vi "Unit Test.vi"() -> ()   [LabVIEW 2018]
uses:
  Force Test Stand.lvclass
  Force Test Stand.lvclass/Force Test Stand.ctl
panel:
  out "error out":errorcluster
  in  "error in (no error)":errorcluster
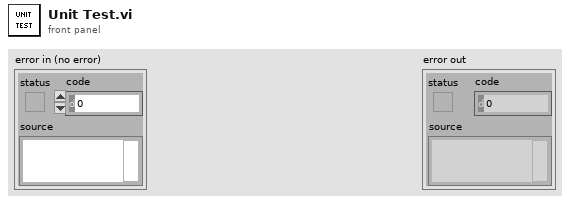
[diagram p1: front panel]
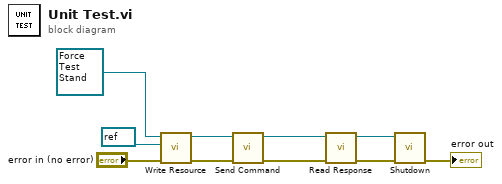
[diagram p0: block diagram]
diagram:
  n1 = call "Write Resource.vi"("error in (no error)"="error in (no error)", "Resource"=refnum<visa-resource-name> refnum, "Force Test Stand in"=refnum<class "Force Test Stand.lvclass"> refnum) -> ("error out"=w1:errorcluster, "Force Test Stand out"=w2:refnum<class "Force Test Stand.lvclass">)  [unwired: 7 in]
  n2 = call-dynamic "Send Command.vi"("error in (no error)"=w1, "Force Test Stand in"=w2) -> ("error out"=w5:errorcluster, "Force Test Stand out"=w6:refnum<class "Force Test Stand.lvclass">)  [unwired: 8 in]
  n3 = call-dynamic "Read Response.vi"("error in (no error)"=w5, "Force Test Stand in"=w6) -> ("error out"=w3:errorcluster, "Force Test Stand out"=w4:refnum<class "Force Test Stand.lvclass">)  [unwired: 8 in]
  n4 = call "Shutdown.vi"("error in (no error)"=w3, "Force Test Stand in"=w4) -> ("error out"=→"error out":errorcluster)  [unwired: 8 in, 1 out]
